vi "AIMeasureAudio.vi"(0 "Physical Channel":tag="DAQ/ai0", 1 "Max Voltage":dbl=10.0, 2 "Terminal Configuration":i32(ring)=-1 items=["default"=-1, "RSE"=10083, "NRSE"=10078, "Differential"=10106, "Pseudodifferential"=12529], 3 "Min Voltage":dbl=-10.0, 4 "Sample Rate":dbl=96000.0, 5 "Number of Samples":i32=19200, 7 "advanced search":T1={"approx freq. (optional)"=-1.0, "search (+/- % of Fsampl.)"=5.0} {"search (+/- % of Fsampl.)" format="%0.2p"; "approx freq. (optional)" format="%0.2p"}, 9 "highest harmonic":i32=5) -> (14 "RMS (V)":dbl[](array[numeric]) format="%.2p", 15 "Detected Fundamental Frequencies (Hz)":dbl[](array[numeric]) format="%.2p", 17 "THD (%)":dbl[](array[numeric]) format="%.2p", 19 "error out":errorcluster)   [LabVIEW 2012]
uses:
  <vilib>/DAQmx/read.llb/DAQmx Read (Analog 1D Wfm NChan NSamp).vi
  <vilib>/DAQmx/create/channels.llb/DAQmx Create Channel (AI-Voltage-Basic).vi
  <vilib>/DAQmx/configure/timing.llb/DAQmx Timing (Sample Clock).vi
  <vilib>/measure/madcrms.llb/Basic Averaged DC-RMS for N Chan.vi
  <vilib>/measure/matone.llb/Harmonic Distortion Analyzer N Chan.vi
  <vilib>/DAQmx/miscellaneous.llb/DAQmx Fill In Error Info.vi
  <vilib>/measure/NI_MAPro.lvlib
panel:
  out "Waveform Graph":waveform(dbl)[](graph)
  # "Channel Settings"
  # "Acquired Data"
  # "Timing Settings"
  # "Results"
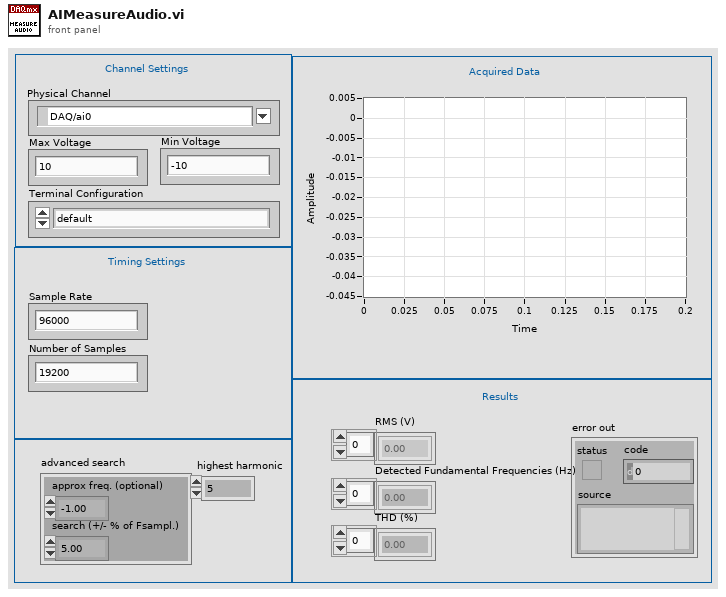
[diagram p1: front panel]
types:
  T1 = cluster{"approx freq. (optional)":dbl, "search (+/- % of Fsampl.)":dbl}
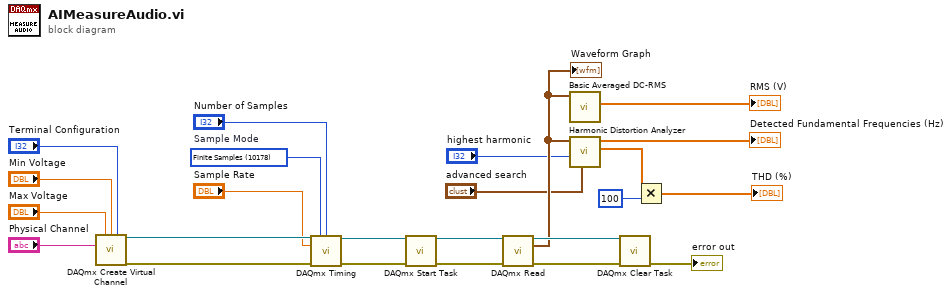
[diagram p0: block diagram]
diagram:
  w24 = 10178 items=["Finite Samples"=10178, "Continuous Samples"=10123, "Hardware Timed Single Point"=12522]  # Sample Mode
  n1 = call-poly <vilib>:"DAQmx Create Virtual Channel.vi"("maximum value"="Max Voltage", "minimum value"="Min Voltage", "input terminal configuration"="Terminal Configuration", "physical channels"="Physical Channel") -> ("task out"=w22:refnum<k21>, "error out"=w23:errorcluster)  [unwired: 10 in]
  n2 = call-poly <vilib>:"DAQmx Timing.vi"("task/channels in"=w22, "sample mode"=w24, "samples per channel"="Number of Samples", "rate"="Sample Rate", "error in"=w23) -> ("task out"=w11:refnum<k21>, "error out"=w10:errorcluster)  [unwired: 9 in]
  n3 = call <vilib>:"DAQmx Start Task.vi"("task/channels in"=w11, "error in"=w10) -> ("task out"=w21:refnum<k21>, "error out"=w20:errorcluster)  [unwired: 12 in]
  n4 = call-poly <vilib>:"DAQmx Read.vi"("task/channels in"=w21, "error in"=w20) -> ("task out"=w19:refnum<k21>, "data"=w8:waveform(dbl)[], "error out"=w18:errorcluster)  [unwired: 11 in]
  "Waveform Graph" <- w8
  n5 = call-poly <vilib>:"Basic Averaged DC-RMS.vi"("signals in"=w8) -> ("RMS values"=→"RMS (V)":dbl[])  [unwired: 7 in, 3 out]
  n6 = call-poly <vilib>:"Harmonic Distortion Analyzer.vi"("advanced search"="advanced search", "highest harmonic"="highest harmonic", "signals in"=w8) -> ("THD"=w5:dbl[], "detected fundamental frequencies"=→"Detected Fundamental Frequencies (Hz)":dbl[])  [unwired: 3 in, 4 out]
  n7 = call <vilib>:"DAQmx Clear Task.vi"("task in"=w19, "error in"=w18) -> ("error out"=→"error out":errorcluster)  [unwired: 13 in]
  n8 = Multiply(x=w5, y=100 ("THD")) -> (x*y=→"THD (%)":dbl[])
